vi "rejectCommand.vi"(8 "error in (no error)":errorcluster, 10 "InternalCommandId.lvclass":refnum<class "InternalCommandId.lvclass">, 11 "ElectrometerController in":refnum<class "ElectrometerController.lvclass">) -> (0 "error out":errorcluster, 3 "ElectrometerController out":refnum<class "ElectrometerController.lvclass">)   [LabVIEW 2016, in "ElectrometerController.lvclass"]
uses:
  ElectrometerController.lvclass
  InternalCommandId/InternalCommandId.lvclass
  ts_electrometeruserevents/Typedefs/CommandValue.ctl
  ElectrometerController.lvclass/ElectrometerController.ctl
  ts_electrometeruserevents/PubSubDataEvent/PubSubDataEvent.lvclass
  ts_electrometeruserevents/Typedefs/ElectrometerTypedefs.lvlib
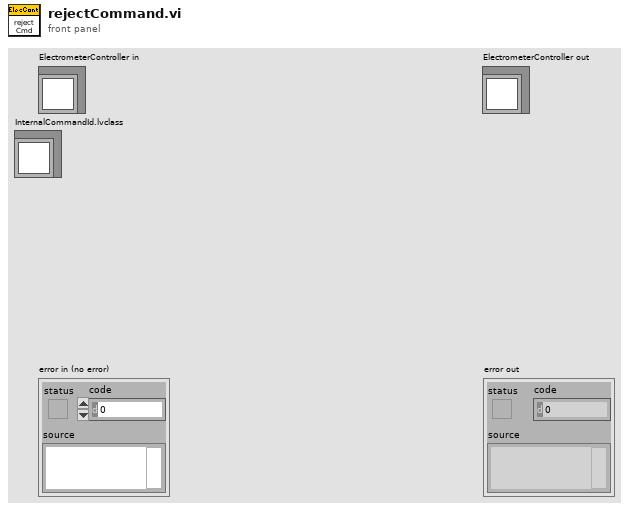
[diagram p1: front panel]
types:
  T1 = typedef "ElectrometerTypedefs.lvlib/CommandValue.ctl" = enum16{"N/A", "Disable", "Enable", "Exit", "GoToStandby", "OnHeartbeat", "OnIncomingMessagingError", "OnInterrupt", "Start", "SetDigitalFilter", "StartScan", "StartScanDt", "StartScanReachIntensity", "StopScan", "SetIntegrationTime", "PerformZeroCalib", "SetRange", "SetMode", "Power"}
  T2 = cluster{"error":i32, "result":string, "ack":i32, "cmdSeqNum":i32, "CommandValue":T1}
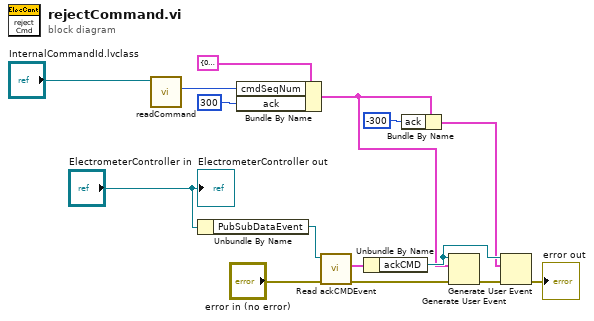
[diagram p0: block diagram]
diagram:
  n1 = call "readCommand.vi"("InternalCommandId in"="InternalCommandId.lvclass") -> ("CommandID"=w9:i32)  [unwired: 7 in, 3 out]
  n2 = Unbundle By Name("ElectrometerController in") -> ("PubSubDataEvent"=w7:refnum<class "PubSubDataEvent.lvclass">)
  n3 = Bundle By Name(cluster=T2 {"error"=0, "result"="", "ack"=0, "cmdSeqNum"=0, "CommandValue"=enum."N/A"} ("event data"), "cmdSeqNum"=w9, "ack"=300) -> (w3:T2)
  n4 = call-dynamic "Read ackCMDEvent.vi"("error in (no error)"="error in (no error)", "PubSubDataEvent in"=w7) -> ("error out"=w14:errorcluster, "ackCMDEvent"=w12:cluster{"ackCMD":refnum<user-event>})  [unwired: 7 in, 1 out]
  n5 = Unbundle By Name(w12) -> ("ackCMD"=w4:refnum<user-event>)
  n6 = Bundle By Name(cluster=w3, "ack"=-300) -> (w1:T2)
  n7 = Generate User Event(user event=w4, event data cluster=w3, error in=w14) -> (error out=w6:errorcluster)  [unwired: 1 in, 1 out]
  n8 = Generate User Event(user event=w4, event data cluster=w1, error in=w6) -> (error out=→"error out":errorcluster)  [unwired: 1 in, 1 out]
  "ElectrometerController out" <- "ElectrometerController in"
